vi "APS stop move multi.vi"(8 "error in (no error)":errorcluster caption="错误输入（无错误）", 10 "Axis_ID_Array":i32[](array[numeric]), 11 "Dimension":i32) -> (0 "error out":errorcluster caption="错误输出", 2 "Axis_ID_Array 2":i32[](array[numeric]), 3 "function return":i32)   [LabVIEW 2012, in "APS168.lvlib"]
doc: "I32 FNTYPE APS_stop_move_multi( I32 Dimension, I32 *Axis_ID_Array );"
uses:
  APS168.lvlib
  APS168.dll
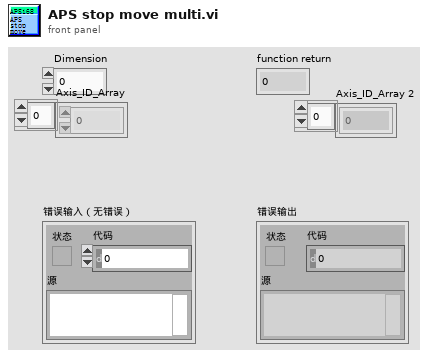
[diagram p1: front panel]
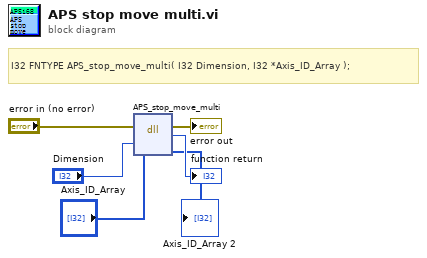
[diagram p0: block diagram]
diagram:
  # "I32 FNTYPE APS_stop_move_multi( I32 Dimension, I32 *Axis_ID_Array );"
  n1 = dll-call lib="PTH1*abs E\t冲压机运动204cAPS168.*" fn="APS_stop_move_multi"(error in="error in (no error)", "Dimension"="Dimension", "Axis_ID_Array"="Axis_ID_Array") -> (error out=→"error out":errorcluster, "return type"=→"function return":i32, "Axis_ID_Array"=→"Axis_ID_Array 2":i32[])  [unwired: 3 in, 1 out]
